vi "Read Teller.vi"(11 "Stopped Msg in":refnum<class "--Stopped Msg.lvclass">) -> (2 "Teller":refnum<class "Teller.lvclass">)   [LabVIEW 2025, in "jettl.lvlib" / "Stopped jettl Msg.lvlib" / "--Stopped Msg.lvclass"]
uses:
  --Stopped Msg.lvclass
  Teller/Teller.lvclass
  --Stopped Msg.lvclass/--Stopped Msg.ctl
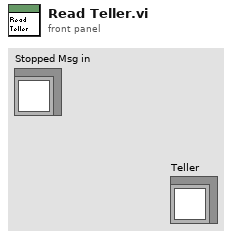
[diagram p1: front panel]
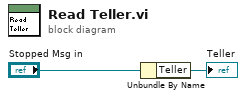
[diagram p0: block diagram]
diagram:
  n1 = Unbundle By Name("Stopped Msg in") -> ("Teller"=→"Teller":refnum<class "Teller.lvclass">)
